vi "mqttReadByteQuantity.vi"(0 "rxTelegram in":u8[](array[numeric]) format="%02x", 11 "error in (no error)":errorcluster) -> (6 "remainingLength":i32, 8 "lengthByteQuantity":i32, 15 "error out":errorcluster)   [LabVIEW 2020, in "MQTT Client.lvclass"]
uses:
  MQTT Client.lvclass
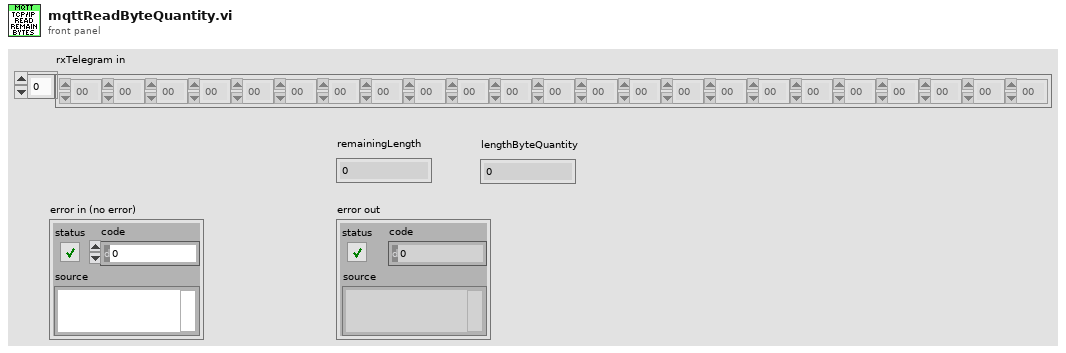
[diagram p1: front panel]
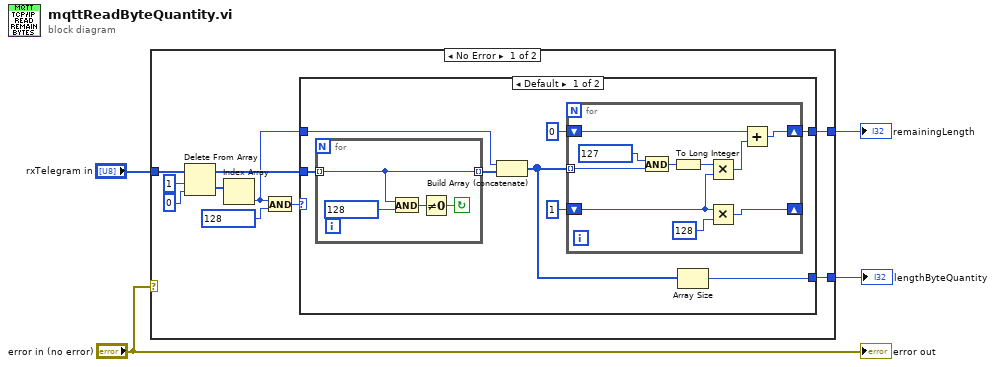
[diagram p0: block diagram]
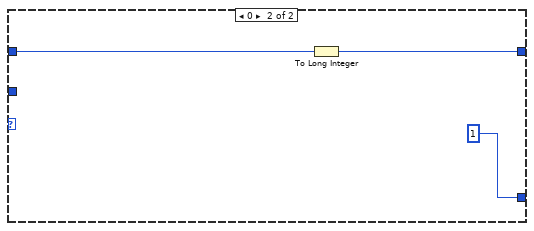
[diagram p2: hidden frame]
diagram:
  n1 = case shown="No Error" "error in (no error)" {
    tunnel: [w12 _] -> w4
    tunnel: "rxTelegram in" -> [w11 _]
    tunnel: [w5 _] -> w1
    frame No Error {
      n2 = Delete From Array(array=w11, length=1, index=0) -> (deleted portion=w8:u8[], array with subset deleted=w10:u8[])
      n3 = Index Array(array=w8) -> (element=w7:u8)  [unwired: 1 in]
      n4 = And(x=w7, y=u8 128) -> (x .and. y?=w13:u8)
      n5 = case shown="Default" w13 {
        tunnel: [w20 w39] -> w12
        tunnel: w10 -> [w19 _]
        tunnel: w7 -> [w17 w38]
        tunnel: [w15 1] -> w5
        frame Default {
          n6 = for {
            tunnel: [w23] -> w18 mode=indexing
            tunnel: w19 -> [w23] mode=indexing
            stop <- w24 continue-if-true
            n7 = And(x=w23, y=u8 128) -> (x .and. y?=w25:u8)
            n8 = Not Equal To 0?(x=w25) -> (x != 0?=w24:bool)
          }
          n9 = Build Array (concatenate)(w17, w18) -> (w16:u8[])
          n10 = for {
            tunnel: w16 -> [w36] mode=indexing
            shift-right: [w32] -> w20
            shift-left: 0 -> [w31]
            shift-right: [w27] -> _
            shift-left: 1 -> [w28]
            n11 = And(x=u8 127 ("y"), y=w36) -> (x .and. y?=w34:u8)
            n12 = To Long Integer(number=w34) -> (32bit integer=w33:i32)
            n13 = Multiply(x=w33, y=w28) -> (x*y=w30:i32)
            n14 = Multiply(x=w28, y=128 ("x")) -> (x*y=w27:i32)
            n15 = Add(x=w31, y=w30) -> (x+y=w32:i32)
          }
          n16 = Array Size(array=w16) -> (size(s)=w15:i32)
        }
        frame 0 {
          n17 = To Long Integer(number=w38) -> (32bit integer=w39:i32)
        }
      }
    }
    frame Error {
    }
  }
  "remainingLength" <- w4
  "lengthByteQuantity" <- w1
  "error out" <- "error in (no error)"
